vi "velosterstack384.vi"(11 "VELO_384":T1 {"hash" format="%016x"}) -> ()   [LabVIEW 2015]
uses:
  G_SEN.vi
panel:
  out "XY Graph":cluster{"X":dbl, "Y":dbl}[](graph)
  out "d":dbl[](array[numeric])
  out "Z":dbl[](array[numeric])
  out "Y":dbl[](array[numeric])
  out "X":dbl[](array[numeric])
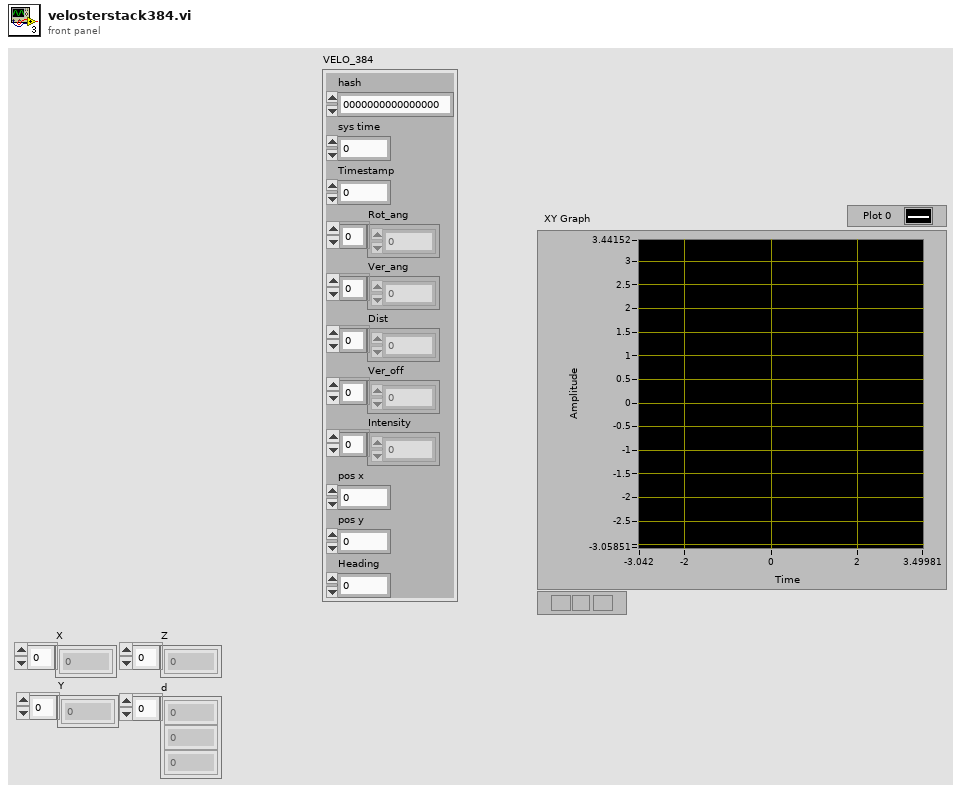
[diagram p1: front panel]
types:
  T1 = cluster{"hash":i64, "sys time":i64, "Timestamp":u32, "Rot_ang":dbl[], "Ver_ang":dbl[], "Dist":dbl[], "Ver_off":dbl[], "Intensity":u8[], "pos x":dbl, "pos y":dbl, "Heading":dbl}
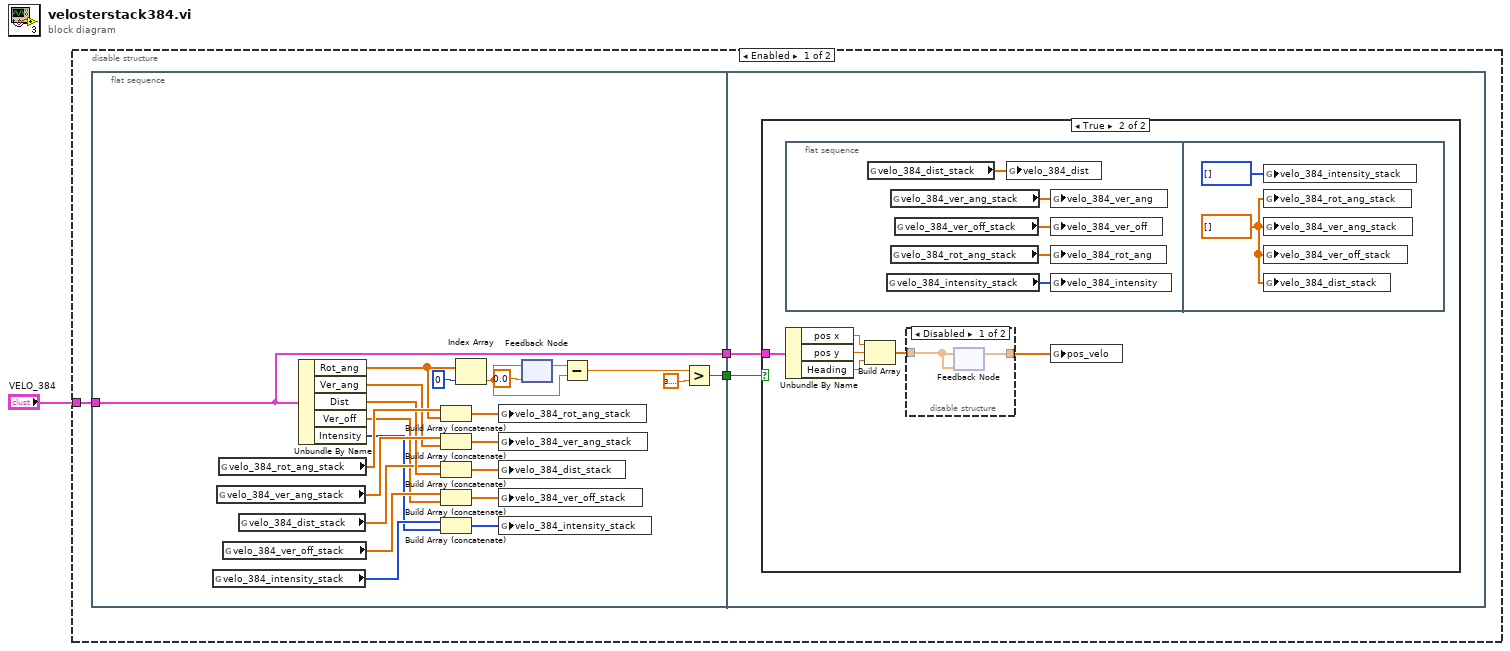
[diagram p0: block diagram]
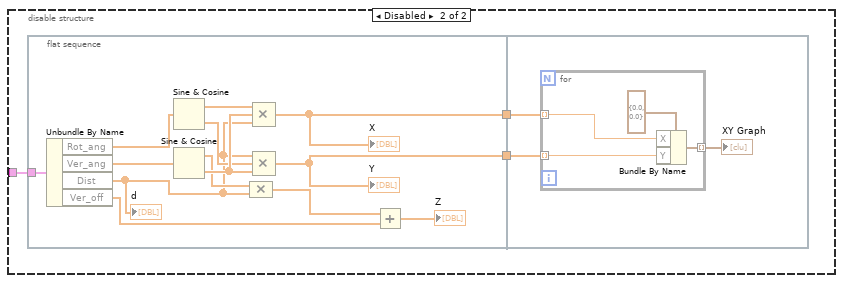
[diagram p4: hidden frame]
diagram:
  n1 = disable-structure shown="Enabled" {
    disable-tunnel: "VELO_384" -> [w3 w48]
    frame Enabled {
      n2 = flat-sequence {
        tunnel: [w13] -> w4
        tunnel: w3 -> [w13]
        tunnel: [w7] -> w2
        tunnel: w4 -> [w29]
        tunnel: w2 -> [w28]
        frame #0 {
          n3 = global read "G_SEN.vi" "velo_384_intensity_stack"() -> (w17:u8[])
          n4 = global read "G_SEN.vi" "velo_384_ver_ang_stack"() -> (w24:dbl[])
          n5 = global read "G_SEN.vi" "velo_384_rot_ang_stack"() -> (w27:dbl[])
          n6 = global read "G_SEN.vi" "velo_384_ver_off_stack"() -> (w19:dbl[])
          n7 = global read "G_SEN.vi" "velo_384_dist_stack"() -> (w22:dbl[])
          n8 = Unbundle By Name(w13) -> ("Rot_ang"=w12:dbl[], "Ver_ang"=w14:dbl[], "Dist"=w23:dbl[], "Ver_off"=w18:dbl[], "Intensity"=w15:u8[])
          n9 = Build Array (concatenate)(w27, w12) -> (w26:dbl[])
          n10 = Build Array (concatenate)(w24, w14) -> (w25:dbl[])
          n11 = Build Array (concatenate)(w22, w23) -> (w21:dbl[])
          n12 = Build Array (concatenate)(w19, w18) -> (w20:dbl[])
          n13 = Build Array (concatenate)(w17, w15) -> (w16:u8[])
          n14 = Index Array(array=w12, index=0) -> (element=w5:dbl)
          n15 = global write "G_SEN.vi" "velo_384_rot_ang_stack"(w26) -> ()
          n16 = global write "G_SEN.vi" "velo_384_ver_ang_stack"(w25) -> ()
          n17 = global write "G_SEN.vi" "velo_384_dist_stack"(w21) -> ()
          n18 = global write "G_SEN.vi" "velo_384_ver_off_stack"(w20) -> ()
          n19 = global write "G_SEN.vi" "velo_384_intensity_stack"(w16) -> ()
          n20 = feedback-in #1(w5) -> ()
          n21 = feedback #1(0.0) -> (w6:dbl)
          n22 = Subtract(x=w6, y=w5) -> (x-y=w9:dbl)
          n23 = Greater?(x=w9, y=3.141592653589793) -> (0:w7:bool)
        }
        frame #1 {
          n24 = case shown="True" w28 {
            tunnel: w29 -> [_ w30]
            frame False {
            }
            frame True {
              n25 = flat-sequence {
                frame #0 {
                  n26 = global read "G_SEN.vi" "velo_384_dist_stack"() -> (w40:dbl[])
                  n27 = global read "G_SEN.vi" "velo_384_intensity_stack"() -> (w37:u8[])
                  n28 = global read "G_SEN.vi" "velo_384_ver_ang_stack"() -> (w38:dbl[])
                  n29 = global read "G_SEN.vi" "velo_384_rot_ang_stack"() -> (w39:dbl[])
                  n30 = global read "G_SEN.vi" "velo_384_ver_off_stack"() -> (w36:dbl[])
                  n31 = global write "G_SEN.vi" "velo_384_dist"(w40) -> ()
                  n32 = global write "G_SEN.vi" "velo_384_ver_ang"(w38) -> ()
                  n33 = global write "G_SEN.vi" "velo_384_ver_off"(w36) -> ()
                  n34 = global write "G_SEN.vi" "velo_384_rot_ang"(w39) -> ()
                  n35 = global write "G_SEN.vi" "velo_384_intensity"(w37) -> ()
                }
                frame #1 {
                  w41 = dbl[] [] ("velo_384_dist_stack")
                  n36 = global write "G_SEN.vi" "velo_384_intensity_stack"(u8[] [] ("velo_384_dist_stack")) -> ()
                  n37 = global write "G_SEN.vi" "velo_384_rot_ang_stack"(w41) -> ()
                  n38 = global write "G_SEN.vi" "velo_384_ver_ang_stack"(w41) -> ()
                  n39 = global write "G_SEN.vi" "velo_384_ver_off_stack"(w41) -> ()
                  n40 = global write "G_SEN.vi" "velo_384_dist_stack"(w41) -> ()
                }
              }
              n41 = Unbundle By Name(w30) -> ("pos x"=w35:dbl, "pos y"=w34:dbl, "Heading"=w33:dbl)
              n42 = Build Array(w35, w34, w33) -> (w32:dbl[])
              n43 = disable-structure shown="Disabled" {
                disable-tunnel: w32 -> [w44 w45]
                disable-tunnel: [w43 w45] -> w31
                frame Disabled {
                  n44 = feedback #2(w44) -> (w43:dbl[])
                  n45 = feedback-in #2(w44) -> ()
                }
                frame Enabled {
                }
              }
              n46 = global write "G_SEN.vi" "pos_velo"(w31) -> ()
            }
          }
        }
      }
    }
    frame Disabled {
      n47 = flat-sequence {
        tunnel: w48 -> [w61]
        tunnel: [w50] -> w47
        tunnel: [w49] -> w46
        tunnel: w47 -> [w64]
        tunnel: w46 -> [w63]
        frame #0 {
          n48 = Unbundle By Name(w61) -> ("Rot_ang"=w54:dbl[], "Ver_ang"=w53:dbl[], "Dist"=w52:dbl[], "Ver_off"=w51:dbl[])
          "d" <- w52
          n49 = Sine & Cosine(0:w54) -> (1:w59:dbl[], 2:w58:dbl[])
          n50 = Sine & Cosine(0:w53) -> (1:w57:dbl[], 2:w60:dbl[])
          n51 = Compound Arithmetic op=MULTIPLY(w57, w52) -> (w56:dbl[])
          n52 = Compound Arithmetic op=MULTIPLY(w59, w60, w52) -> (w50:dbl[])
          "X" <- w50
          n53 = Compound Arithmetic op=MULTIPLY(w52, w58, w60) -> (w49:dbl[])
          "Y" <- w49
          n54 = Add(x=w56, y=w51) -> (x+y=→"Z":dbl[])
        }
        frame #1 {
          n55 = for {
            tunnel: w64 -> [w67] mode=indexing
            tunnel: w63 -> [w66] mode=indexing
            tunnel: [w65] -> w62 mode=indexing
            n56 = Bundle By Name(cluster=cluster{"X":dbl, "Y":dbl} {"X"=0.0, "Y"=0.0}, "X"=w67, "Y"=w66) -> (w65:cluster{"X":dbl, "Y":dbl})
          }
          "XY Graph" <- w62
        }
      }
    }
  }
